vi "user process.vi"(8 "error in":errorcluster, 10 "Model State In":T1, 11 "Parameters to process":T3) -> (0 "error out":errorcluster, 2 "Model State Out":T1, 3 "Results from processing":T2)   [LabVIEW 2013, in "Temperature Chamber Model runtime.lvclass"]
uses:
  Temperature Chamber Model runtime.lvclass
  parameter user data.ctl
  result user data.ctl
  model state.ctl
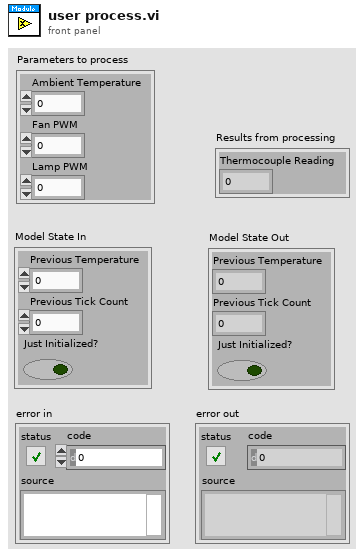
[diagram p1: front panel]
types:
  T1 = typedef "Temperature Chamber Model runtime.lvclass/model state.ctl" = cluster{"Previous Temperature":dbl, "Previous Tick Count":u32, "Just Initialized?":bool}
  T2 = typedef "Temperature Chamber Model runtime.lvclass/result user data.ctl" = cluster{"Thermocouple Reading":dbl}
  T3 = typedef "Temperature Chamber Model runtime.lvclass/parameter user data.ctl" = cluster{"Ambient Temperature":dbl, "Fan PWM":dbl, "Lamp PWM":dbl}
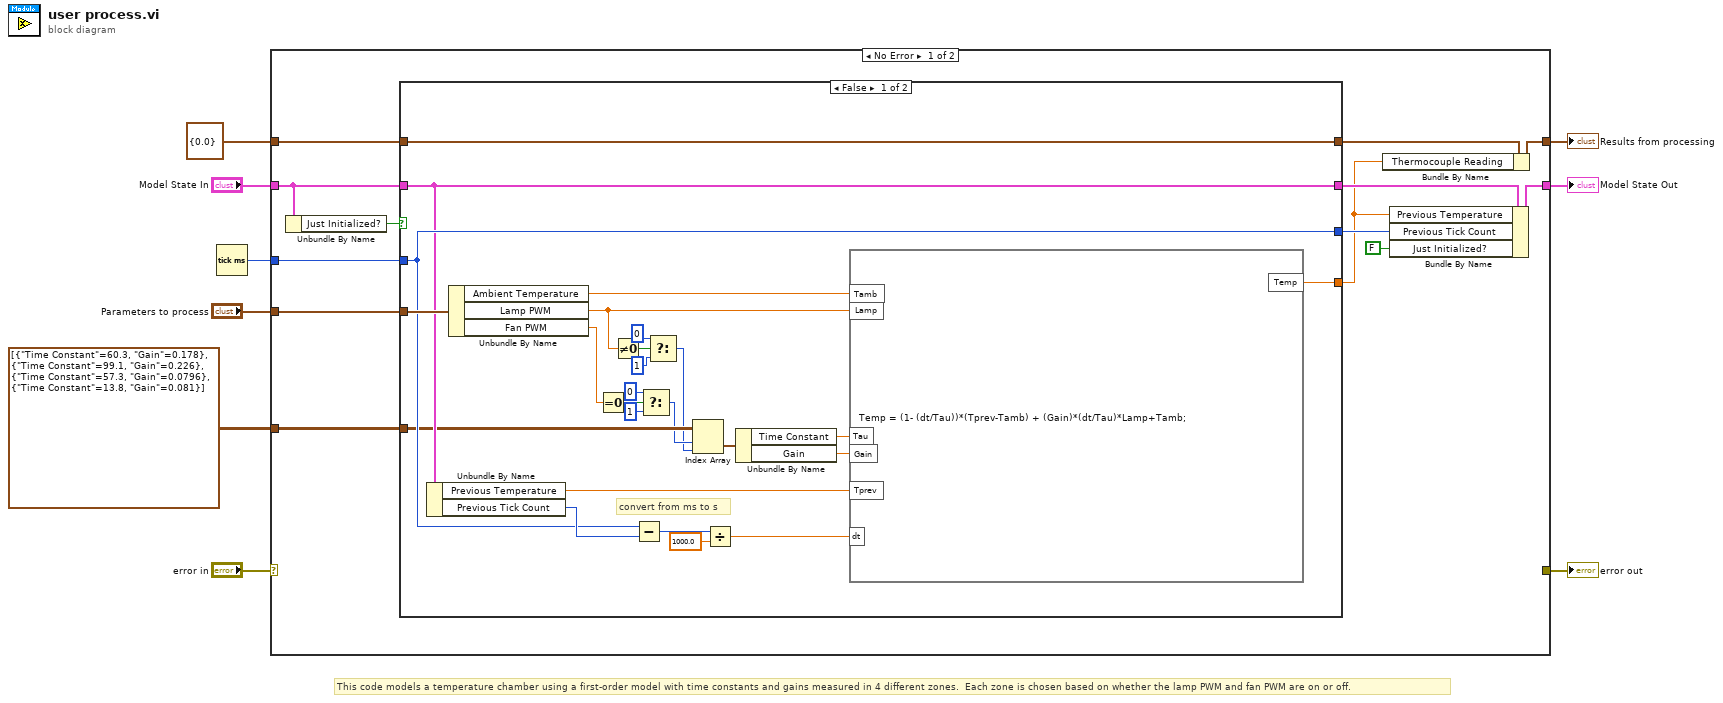
[diagram p0: block diagram]
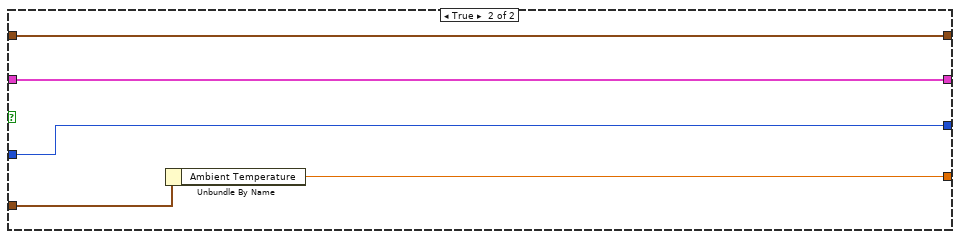
[diagram p2: hidden frame]
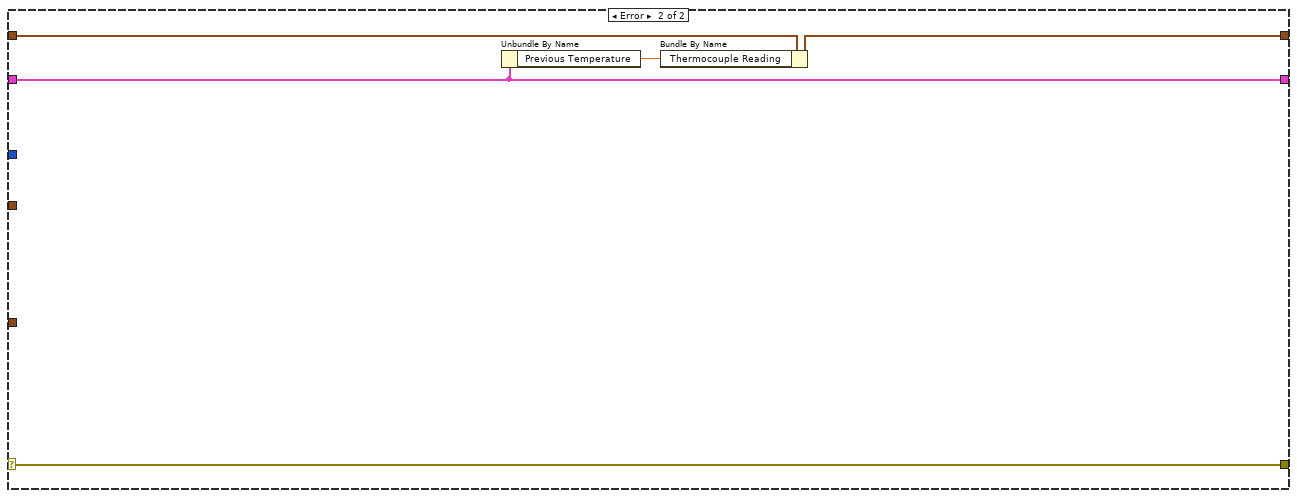
[diagram p3: hidden frame]
diagram:
  # "This code models a temperature chamber using a first-order model with time constants and gains measured in 4 different zones.  Each zone is chosen based on whether the lamp PWM and fan PWM are on or off."
  n1 = Tick Count (ms)() -> (millisecond timer value=w5:u32)
  n2 = case shown="No Error" "error in" {
    selector: "error in" -> [_ w57]
    tunnel: "Model State In" -> [w15 w54]
    tunnel: "Parameters to process" -> [w21 _]
    tunnel: [_ w57] -> w6
    tunnel: w5 -> [w16 _]
    tunnel: [w17 w54] -> w4
    tunnel: T2 {"Thermocouple Reading"=0.0} ("Results from processing") -> [w14 w56]
    tunnel: [w12 w55] -> w2
    tunnel: cluster{"Time Constant":dbl, "Gain":dbl}[][] [[{"Time Constant"=60.3, "Gain"=0.178}, {"Time Constant"=99.1, "Gain"=0.226}], [{"Time Constant"=57.3, "Gain"=0.0796}, {"Time Constant"=13.8, "Gain"=0.081}]] -> [w10 _]
    frame No Error {
      n3 = Unbundle By Name(w15) -> ("Just Initialized?"=w22:bool)
      n4 = case shown="False" w22 {
        tunnel: w21 -> [w47 w52]
        tunnel: [w37 w50] -> w20
        tunnel: [w38 w51] -> w11
        tunnel: [w44 w48] -> w19
        tunnel: w16 -> [w44 w48]
        tunnel: w15 -> [w37 w50]
        tunnel: w14 -> [w40 w49]
        tunnel: [w40 w49] -> w13
        tunnel: w10 -> [w36 _]
        frame False {
          # "convert from ms to s"
          n5 = Unbundle By Name(w37) -> ("Previous Temperature"=w46:dbl, "Previous Tick Count"=w45:u32)
          n6 = Unbundle By Name(w47) -> ("Ambient Temperature"=w39:dbl, "Lamp PWM"=w29:dbl, "Fan PWM"=w34:dbl)
          n7 = Equal To 0?(x=w34) -> (x = 0?=w33:bool)
          n8 = Not Equal To 0?(x=w29) -> (x != 0?=w26:bool)
          n9 = Subtract(x=w44, y=w45) -> (x-y=w42:u32)
          n10 = Select(t=u32 0, s=w33, f=u32 1) -> (s? t:f=w30:u32)
          n11 = Select(t=u32 0, s=w26, f=u32 1) -> (s? t:f=w25:u32)
          n12 = Index Array(array=w36, index (row)=w30, index (col)=w25) -> (element=w35:cluster{"Time Constant":dbl, "Gain":dbl})
          n13 = Divide(x=w42, y=1000.0) -> (x/y=w41:dbl)
          n14 = Unbundle By Name(w35) -> ("Time Constant"=w23:dbl, "Gain"=w24:dbl)
          n15 = formula code="Temp = (1- (dt/Tau))*(Tprev-Tamb) + (Gain)*(dt/Tau)*Lamp+Tamb;"("dt"=w41, "Tau"=w23, "Tprev"=w46, "Lamp"=w29, "Tamb"=w39, "Gain"=w24) -> ("Temp"=w38:dbl)
        }
        frame True {
          n16 = Unbundle By Name(w52) -> ("Ambient Temperature"=w51:dbl)
        }
      }
      n17 = Bundle By Name(cluster=w13, "Thermocouple Reading"=w11) -> (w12:T2)
      n18 = Bundle By Name(cluster=w20, "Previous Temperature"=w11, "Previous Tick Count"=w19, "Just Initialized?"=FALSE) -> (w17:T1)
    }
    frame Error {
      n19 = Unbundle By Name(w54) -> ("Previous Temperature"=w53:dbl)
      n20 = Bundle By Name(cluster=w56, "Thermocouple Reading"=w53) -> (w55:T2)
    }
  }
  "error out" <- w6
  "Results from processing" <- w2
  "Model State Out" <- w4
